vi "Correct Aim.vi"(8 "error in":errorcluster, 11 "Image In":T1) -> (0 "error out":errorcluster, 3 "Image Out":T1)   [LabVIEW 2012]
uses:
  <vilib>/vision/Image Controls.llb/IMAQ Image.ctl
  Rec Targeting.vi
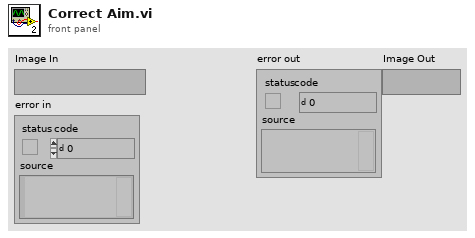
[diagram p1: front panel]
types:
  T1 = typedef "IMAQ Image.ctl" = refnum<image>
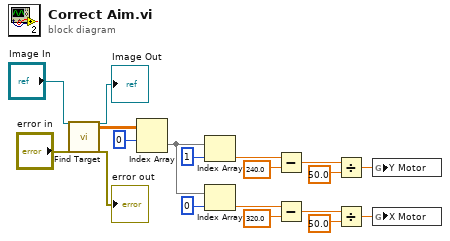
[diagram p0: block diagram]
diagram:
  n1 = call "Find Target.vi"("Image In"="Image In", "error in"="error in") -> ("Image Out"=→"Image Out":T1, "Particle Measurements (Pixels) (Particle Analysis 1)"=w19:dbl[][], "error out"=→"error out":errorcluster)  [unwired: 23 in]
  n2 = Index Array(array=w19, index (row)=0) -> (element=w15:dbl[])  [unwired: 1 in]
  n3 = Index Array(array=w15, index=1) -> (element=w10:dbl)
  n4 = Index Array(array=w15, index=0) -> (element=w12:dbl)
  n5 = Subtract(x=w10, y=240.0) -> (x-y=w8:dbl)
  n6 = Subtract(x=w12, y=320.0) -> (x-y=w6:dbl)
  n7 = Divide(x=w8, y=50.0) -> (x/y=w3:dbl)
  n8 = Divide(x=w6, y=50.0) -> (x/y=w4:dbl)
  n9 = global write "Rec Targeting.vi" "Y Motor"(w3) -> ()
  n10 = global write "Rec Targeting.vi" "X Motor"(w4) -> ()
